vi "Configure Window.vi"(8 "Prompt":string, 9 "Button Label":string, 11 "File Dialog in":refnum<class "File Dialog.lvclass">) -> (3 "File Dialog out":refnum<class "File Dialog.lvclass">)   [LabVIEW 2018, in "File Dialog Actor.lvlib" / "File Dialog.lvclass"]
uses:
  File Dialog.lvclass
  File Dialog.lvclass/File Dialog.ctl
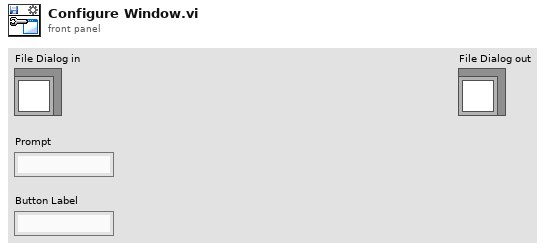
[diagram p1: front panel]
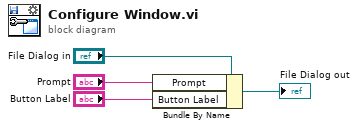
[diagram p0: block diagram]
diagram:
  n1 = Bundle By Name(cluster="File Dialog in", "Prompt"="Prompt", "Button Label"="Button Label") -> (→"File Dialog out":refnum<class "File Dialog.lvclass">)
